vi "Grid_Save_STS_test.vi"(9 "load":u16(ring) items=["numerical_-1V->2V", "numerical_-20mV->20mV", "numerical_-2V->2.2V", "lockin_-20mV->20mV", "lockin_-25mV->25mV", "test", "lockin_highRes_20mV_-20mV", "lockin_slow", "Lock_in_DCA_1.5V->-50mV", "Long_MgPc_lockin_-1->1V", "MgPc_long_lockin", "lockin_slow_-1_2", "MgPc_long_lockin2", "Quick_Lockin"], 10 "stop":bool, 11 "Load":bool) -> (3 "STSTypes []":string[](array[string]))   [LabVIEW 2014]
uses:
  <userlib>/Nanonis Prog Interface V5/Nanonis Prog Interface.lvlib
panel:
  out "loaded":i32
  out "data":T1(array[cluster])
  in  "Save parameters":bool
  in  "Save As":string
  in  "STSparameters":T2 {"End value (V)" min=-10 max=10 format="%#_6p"; "Start value (V)" min=-10 max=10 format="%#_6p"; "End of Sweep"."Z control time (s)" min=0 max=10 step=0.0001 format="%.3p"; "End of Sweep"."End settling time (s)" step=0.0001 format="%.3p"; "Sweep Timing"."Integration time (s)" min=0 max=20 step=0.0001 format="%.3p"; "Sweep Timing"."Settling time (s)" step=0.0001 format="%.3p"; "Sweep Timing"."Max. slew rate (V/s)" format="%.3p"; "Initialization"."Initial settling time (s)" step=0.0001 format="%.3p"; "Initialization"."Z offset (m)" format="%.3p"; "Initialization"."Z averaging time (s)" min=0 max=10 step=0.0001 format="%.3p"; "Amplitude (mod. signal unit)" format="%#_6p"}
  # "make sure\nLockin is activated\nin Advanced Settings"
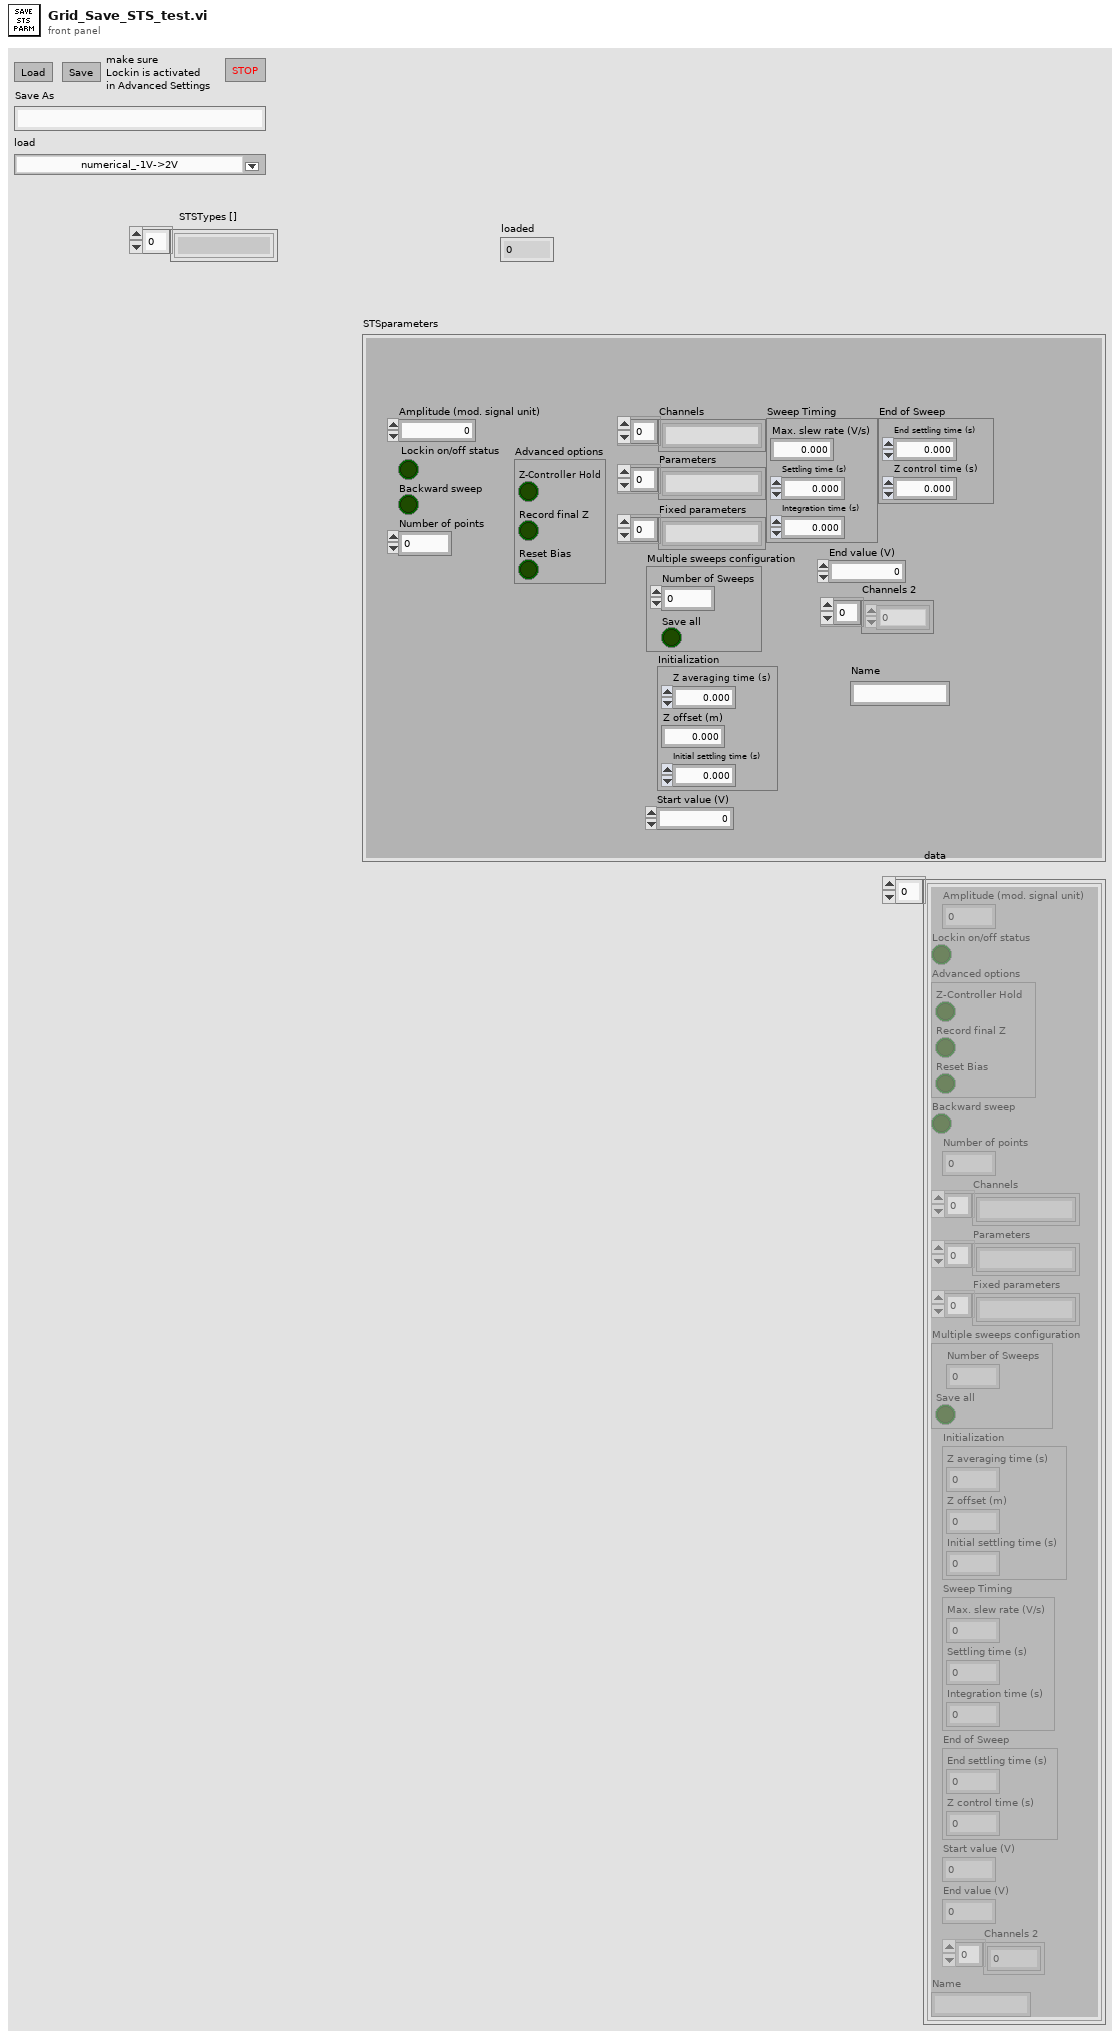
[diagram p1: front panel]
types:
  T1 = cluster{"Amplitude (mod. signal unit)":sgl, "Lockin on/off status":bool, "Advanced options":cluster{"Z-Controller Hold":bool, "Record final Z":bool, "Reset Bias":bool}, "Backward sweep":bool, "Number of points":i32, "Channels":string[], "Parameters":string[], "Fixed parameters":string[], "Multiple sweeps configuration":cluster{"Number of Sweeps":i32, "Save all":bool}, "Initialization":cluster{"Z averaging time (s)":sgl, "Z offset (m)":sgl, "Initial settling time (s)":sgl}, "Sweep Timing":cluster{"Max. slew rate (V/s)":sgl, "Settling time (s)":sgl, "Integration time (s)":sgl}, "End of Sweep":cluster{"End settling time (s)":sgl, "Z control time (s)":sgl}, "Start value (V)":sgl, "End value (V)":sgl, "Channels 2":i32[], "Name":string}[]
  T2 = cluster{"Amplitude (mod. signal unit)":sgl, "Lockin on/off status":bool, "Advanced options":cluster{"Z-Controller Hold":bool, "Record final Z":bool, "Reset Bias":bool}, "Backward sweep":bool, "Number of points":i32, "Channels":string[], "Parameters":string[], "Fixed parameters":string[], "Multiple sweeps configuration":cluster{"Number of Sweeps":i32, "Save all":bool}, "Initialization":cluster{"Z averaging time (s)":sgl, "Z offset (m)":sgl, "Initial settling time (s)":sgl}, "Sweep Timing":cluster{"Max. slew rate (V/s)":sgl, "Settling time (s)":sgl, "Integration time (s)":sgl}, "End of Sweep":cluster{"End settling time (s)":sgl, "Z control time (s)":sgl}, "Start value (V)":sgl, "End value (V)":sgl, "Channels 2":i32[], "Name":string}
  T3 = cluster{"Save all":enum16{"no change", "on", "off"}, "Number of Sweeps (0=no change)":i32}
  T4 = cluster{"Z-Controller Hold":bool, "Record final Z":bool, "Reset Bias":bool}
  T5 = cluster{"Z averaging time (s)":sgl, "Z offset (m)":sgl, "Initial settling time (s)":sgl}
  T6 = cluster{"Max. slew rate (V/s)":sgl, "Settling time (s)":sgl, "Integration time (s)":sgl}
  T7 = cluster{"End settling time (s)":sgl, "Z control time (s)":sgl}
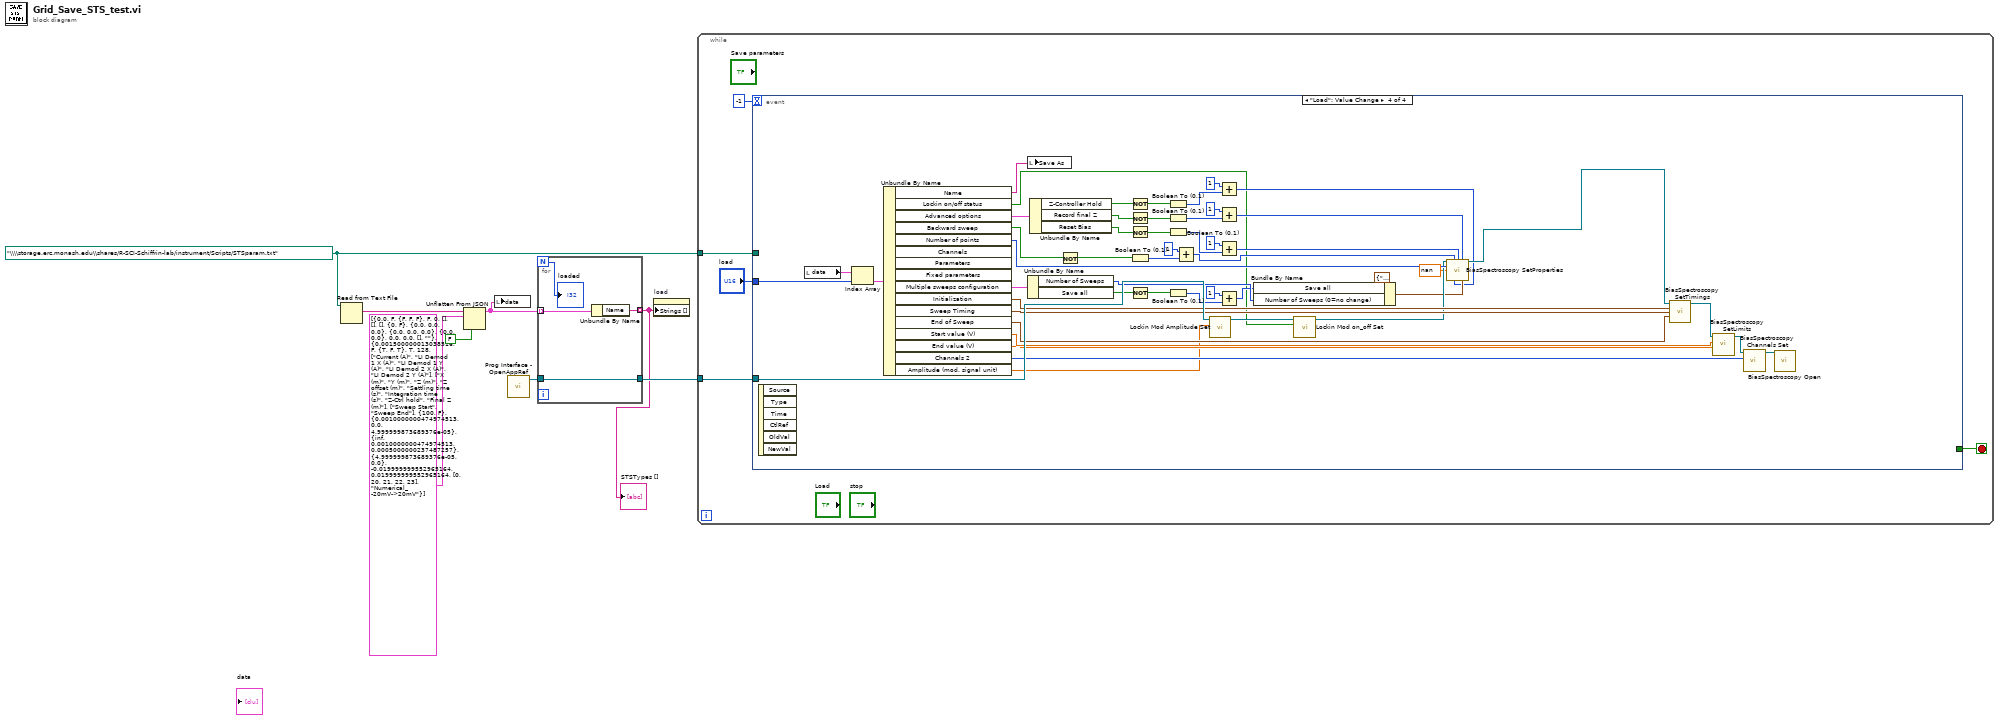
[diagram p0: block diagram]
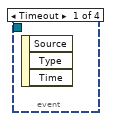
[diagram p2: hidden frame]
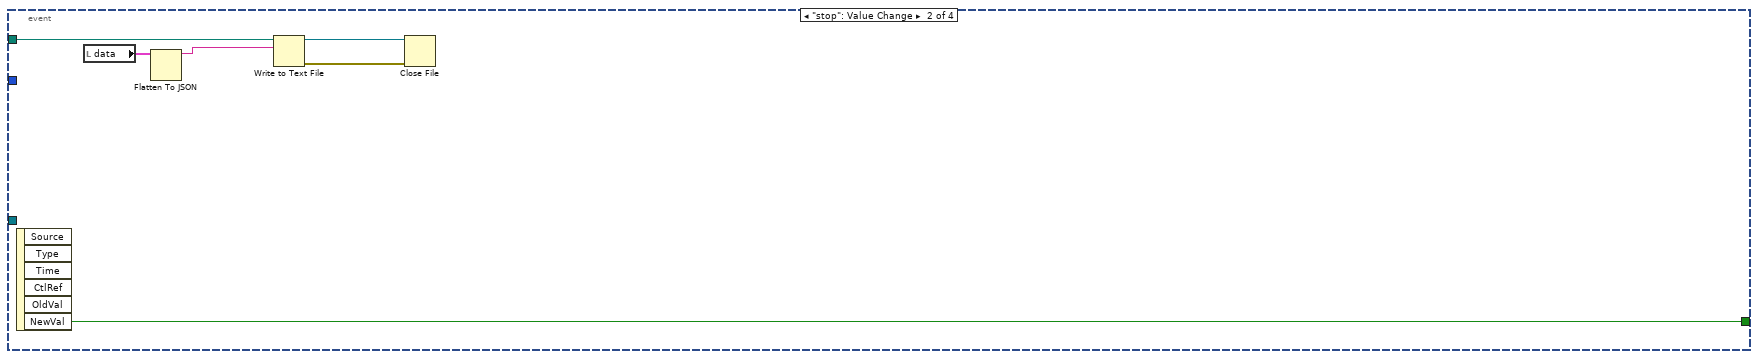
[diagram p3: hidden frame]
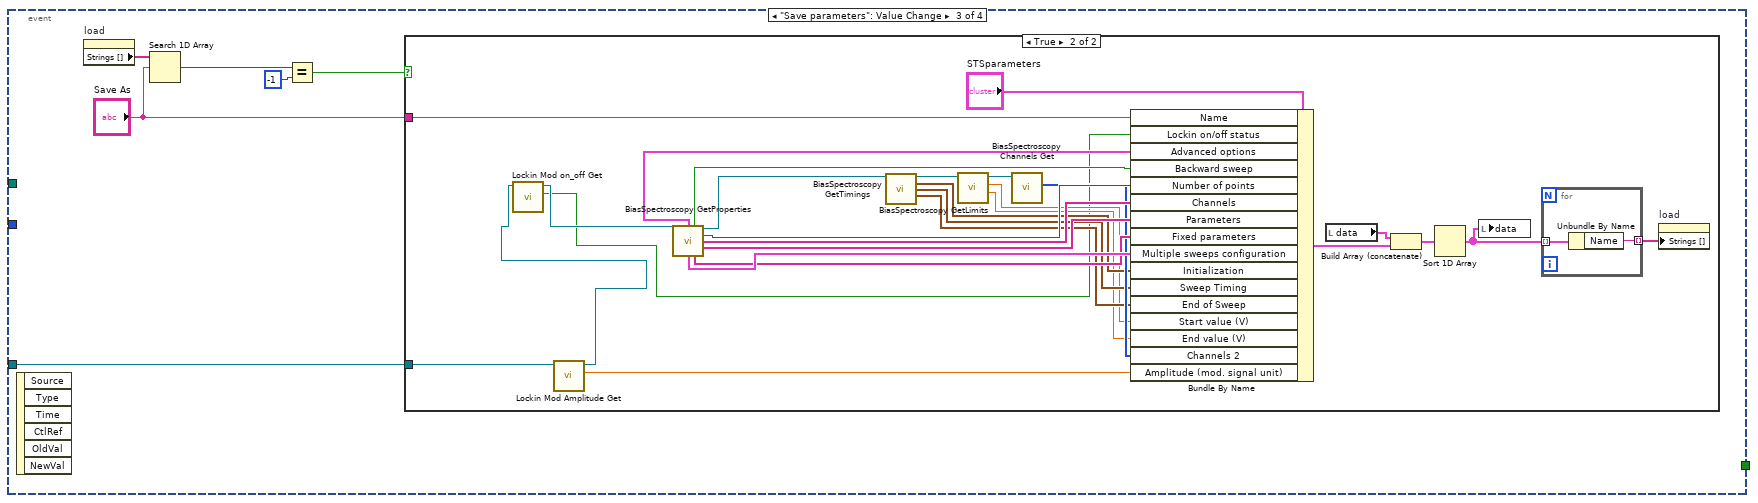
[diagram p4: hidden frame]
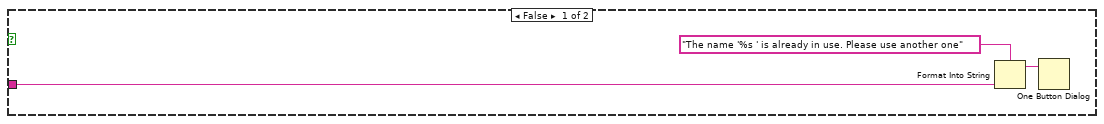
[diagram p5: hidden frame]
diagram:
  w8 = path "\\\\storage.erc.monash.edu\\shares/R-SCI-Schiffrin-lab/instrument/Scripts/STSparam.txt" ("file (use dialog)")
  n1 = Read from Text File(file (use dialog)=w8) -> (text=w7:string)  [unwired: 3 in, 3 out]
  n2 = Unflatten From JSON(JSON string=w7, type and defaults=T1 [{"Amplitude (mod. signal unit)"=0.0, "Lockin on/off status"=FALSE, "Advanced options"={"Z-Controller Hold"=FALSE, "Record final Z"=FALSE, "Reset Bias"=FALSE}, "Backward sweep"=FALSE, "Number of points"=0, "Channels"=[], "Parameters"=[], "Fixed parameters"=[], "Multiple sweeps configuration"={"Number of Sweeps"=0, "Save all"=FALSE}, "Initialization"={"Z averaging time (s)"=0.0, "Z offset (m)"=0.0, "Initial settling time (s)"=0.0}, "Sweep Timing"={"Max. slew rate (V/s)"=0.0, "Settling time (s)"=0.0, "Integration time (s)"=0.0}, "End of Sweep"={"End settling time (s)"=0.0, "Z control time (s)"=0.0}, "Start value (V)"=0.0, "End value (V)"=0.0, "Channels 2"=[], "Name"=""}, {"Amplitude (mod. signal unit)"=0.0015, "Lockin on/off status"=FALSE, "Advanced options"={"Z-Controller Hold"=TRUE, "Record final Z"=FALSE, "Reset Bias"=TRUE}, "Backward sweep"=TRUE, "Number of points"=128, "Channels"=["Current (A)", "LI Demod 1 X (A)", "LI Demod 1 Y (A)", "LI Demod 2 X (A)", "LI Demod 2 Y (A)"], "Parameters"=["X (m)", "Y (m)", "Z (m)", "Z offset (m)", "Settling time (s)", "Integration time (s)", "Z-Ctrl hold", "Final Z (m)"], "Fixed parameters"=["Sweep Start", "Sweep End"], "Multiple sweeps configuration"={"Number of Sweeps"=100, "Save all"=FALSE}, "Initialization"={"Z averaging time (s)"=0.001, "Z offset (m)"=0.0, "Initial settling time (s)"=5e-05}, "Sweep Timing"={"Max. slew rate (V/s)"=inf, "Settling time (s)"=0.001, "Integration time (s)"=0.0005}, "End of Sweep"={"End settling time (s)"=5e-05, "Z control time (s)"=0.0}, "Start value (V)"=-0.02, "End value (V)"=0.02, "Channels 2"=[0, 20, 21, 22, 23], "Name"="Numerical_-20mV->20mV"}] ("data"), default null elements? (F)=FALSE) -> (value=w2:T1)  [unwired: 4 in, 1 out]
  n3 = local write "data"(w2) -> ()
  n4 = call <userlib>:"Prog Interface - OpenAppRef.vi"() -> ("Application reference"=w6:refnum<vi>)  [unwired: 6 in, 1 out]
  n5 = for {
    N -> [w9]
    tunnel: w2 -> [w12] mode=indexing
    tunnel: [w11] -> w1 mode=indexing
    tunnel: w6 -> [w10]
    tunnel: [w10] -> w5
    n6 = Unbundle By Name(w12) -> ("Name"=w11:string)
    "loaded" <- w9
  }
  "STSTypes []" <- w1
  n7 = property on="load" class="Ring (strict)"("Strings []"=w1) -> ()  [unwired: 2 in, 2 out]
  n8 = while {
    tunnel: w5 -> [w17]
    tunnel: w8 -> [w14]
    stop <- w15 stop-if-true
    n9 = event shown="[3] \"Load\": Value Change" {
      selector: _ -> [_ _ _ _]
      dyn-events: _ -> [_ _ _ _]
      timeout: -1 -> [_ _ _ _]
      tunnel: w17 -> [_ _ w29 w111]
      tunnel: "load" -> [_ _ _ w75]
      tunnel: [_ w23 _ _] -> w15
      tunnel: w14 -> [_ w19 _ _]
      event Timeout {
        n10 = event-data() -> ()  [unwired: 1 in, 3 out]
      }
      event "stop": Value Change {
        n11 = event-data() -> ("NewVal"=w23:bool)  [unwired: 1 in, 5 out]
        n12 = local read "data"() -> (w18:T1)
        n13 = Flatten To JSON(anything=w18) -> (JSON string=w22:string)  [unwired: 2 in, 1 out]
        n14 = Write to Text File(file (use dialog)=w19, text=w22) -> (refnum out=w20:refnum<file>, error out=w21:errorcluster)  [unwired: 2 in, 1 out]
        n15 = Close File(refnum=w20, error in=w21) -> ()  [unwired: 2 out]
      }
      event "Save parameters": Value Change {
        n16 = event-data() -> ()  [unwired: 1 in, 6 out]
        n17 = property on="load" class="Ring (strict)"() -> ("Strings []"=w28:string[])  [unwired: 2 in, 2 out]
        n18 = Search 1D Array(1D array=w28, element="Save As") -> (index of element=w26:i32)  [unwired: 1 in]
        n19 = Equal?(x=w26, y=-1) -> (x = y?=w24:bool)
        n20 = case shown="True" w24 {
          tunnel: w29 -> [_ w44]
          tunnel: "Save As" -> [w32 w37]
          frame False {
            n21 = Format Into String(format string="The name '%s ' is already in use. Please use another one", w32) -> (resulting string=w30:string)  [unwired: 2 in, 1 out]
            n22 = One Button Dialog(message=w30) -> ()  [unwired: 1 in, 1 out]
          }
          frame True {
            n23 = call <userlib>:"Lockin Mod Amplitude Get.vi"("Application ref in"=w44) -> ("Amplitude (mod. signal unit)"=w41:sgl, "Application ref out"=w35:refnum<vi>)  [unwired: 8 in, 1 out]
            n24 = call <userlib>:"Lockin Mod on_off Get.vi"("Application ref in"=w35) -> ("Lockin on/off status"=w33:bool, "Application ref out"=w34:refnum<vi>)  [unwired: 8 in, 1 out]
            n25 = call <userlib>:"BiasSpectroscopy GetProperties.vi"("Application ref in"=w34) -> ("Advanced options"=w36:T4, "Backward sweep"=w52:bool, "Application ref out"=w51:refnum<vi>, "Number of points"=w58:i32, "Channels"=w57:string[], "Parameters"=w56:string[], "Multiple sweeps configuration"=w55:cluster{"Number of Sweeps":i32, "Save all":bool}, "Fixed parameters"=w54:string[])  [unwired: 6 in, 1 out]
            n26 = call <userlib>:"BiasSpectroscopy GetTimings.vi"("Application ref in"=w51) -> ("Application ref out"=w59:refnum<vi>, "Initialization"=w50:T5, "Sweep Timing"=w48:T6, "End of Sweep"=w49:T7)  [unwired: 10 in, 1 out]
            n27 = call <userlib>:"BiasSpectroscopy GetLimits.vi"("Application ref in"=w59) -> ("End value (V)"=w46:sgl, "Start value (V)"=w47:sgl, "Application ref out"=w60:refnum<vi>)  [unwired: 5 in, 1 out]
            n28 = call <userlib>:"BiasSpectroscopy Channels Get.vi"("Application ref in"=w60) -> ("Channels"=w53:i32[])  [unwired: 8 in, 2 out]
            n29 = Bundle By Name(cluster="STSparameters", "Name"=w37, "Lockin on/off status"=w33, "Advanced options"=w36, "Backward sweep"=w52, "Number of points"=w58, "Channels"=w57, "Parameters"=w56, "Fixed parameters"=w54, "Multiple sweeps configuration"=w55, "Initialization"=w50, "Sweep Timing"=w48, "End of Sweep"=w49, "Start value (V)"=w47, "End value (V)"=w46, "Channels 2"=w53, "Amplitude (mod. signal unit)"=w41) -> (w45:T2)
            n30 = local read "data"() -> (w42:T1)
            n31 = Build Array (concatenate)(w42, w45) -> (w40:T1)
            n32 = Sort 1D Array(array=w40) -> (sorted array=w39:T1)
            n33 = local write "data"(w39) -> ()
            n34 = for {
              tunnel: w39 -> [w62] mode=indexing
              tunnel: [w61] -> w38 mode=indexing
              n35 = Unbundle By Name(w62) -> ("Name"=w61:string)
            }
            n36 = property on="load" class="Ring (strict)"("Strings []"=w38) -> ()  [unwired: 2 in, 2 out]
          }
        }
      }
      event "Load": Value Change {
        n37 = event-data() -> ()  [unwired: 1 in, 6 out]
        n38 = local read "data"() -> (w113:T1)
        n39 = Index Array(array=w113, index=w75) -> (element=w112:T2)
        n40 = Unbundle By Name(w112) -> ("Name"=w73:string, "Lockin on/off status"=w63:bool, "Advanced options"=w99:T4, "Backward sweep"=w98:bool, "Number of points"=w101:i32, "Multiple sweeps configuration"=w100:cluster{"Number of Sweeps":i32, "Save all":bool}, "Initialization"=w102:T5, "Sweep Timing"=w103:T6, "End of Sweep"=w104:T7, "Start value (V)"=w106:sgl, "End value (V)"=w105:sgl, "Channels 2"=w107:i32[], "Amplitude (mod. signal unit)"=w74:sgl)  [unwired: 3 out]
        n41 = local write "Save As"(w73) -> ()
        n42 = Unbundle By Name(w100) -> ("Number of Sweeps"=w86:i32, "Save all"=w82:bool)
        n43 = Unbundle By Name(w99) -> ("Z-Controller Hold"=w91:bool, "Record final Z"=w90:bool, "Reset Bias"=w87:bool)
        n44 = Not(x=w98) -> (.not. x?=w78:bool)
        n45 = Not(x=w91) -> (.not. x?=w77:bool)
        n46 = Not(x=w90) -> (.not. x?=w80:bool)
        n47 = Not(x=w87) -> (.not. x?=w79:bool)
        n48 = Boolean To (0,1)(Boolean=w78) -> (0, 1=w97:i16)
        n49 = Not(x=w82) -> (.not. x?=w76:bool)
        n50 = Boolean To (0,1)(Boolean=w77) -> (0, 1=w93:i16)
        n51 = Boolean To (0,1)(Boolean=w80) -> (0, 1=w95:i16)
        n52 = Boolean To (0,1)(Boolean=w79) -> (0, 1=w89:i16)
        n53 = Boolean To (0,1)(Boolean=w76) -> (0, 1=w85:i16)
        n54 = Add(x=i16 1, y=w97) -> (x+y=w72:i16)
        n55 = call <userlib>:"Lockin Mod Amplitude Set.vi"("Amplitude (mod. signal unit)"=w74, "Application ref in"=w111) -> ("Application ref out"=w110:refnum<vi>)  [unwired: 8 in, 1 out]
        n56 = Add(x=i16 1, y=w93) -> (x+y=w64:i16)
        n57 = Add(x=i16 1, y=w95) -> (x+y=w65:i16)
        n58 = Add(x=i16 1, y=w89) -> (x+y=w69:i16)
        n59 = Add(x=i16 1, y=w85) -> (x+y=w83:i16)
        n60 = Bundle By Name(cluster=T3 {"Save all"=enum."no change", "Number of Sweeps (0=no change)"=0} ("Multiple sweeps config"), "Save all"=w83, "Number of Sweeps (0=no change)"=w86) -> (w67:T3)
        n61 = call <userlib>:"Lockin Mod on_off Set.vi"("Lockin ON/OFF"=w63, "Application ref in"=w110) -> ("Application ref out"=w71:refnum<vi>)  [unwired: 8 in, 1 out]
        n62 = call <userlib>:"BiasSpectroscopy SetProperties.vi"("Application ref in"=w71, "Backward sweep (no change)"=w72, "Reset Bias (no change)"=w69, "Record final Z position"=w65, "Number of points (0=no change)"=w101, "Z offset (m) (NaN=no change)"=sgl nan, "Z-Controller hold (no change)"=w64, "Multiple sweeps config"=w67) -> ("Application ref out"=w70:refnum<vi>)  [unwired: 6 in, 1 out]
        n63 = call <userlib>:"BiasSpectroscopy SetTimings.vi"("Application ref in"=w70, "Initialization (NaN)"=w102, "Sweep Timing (NaN)"=w103, "End of Sweep (NaN)"=w104) -> ("Application ref out"=w109:refnum<vi>)  [unwired: 10 in, 1 out]
        n64 = call <userlib>:"BiasSpectroscopy SetLimits.vi"("End value (V)"=w105, "Start value (V)"=w106, "Application ref in"=w109) -> ("Application ref out"=w108:refnum<vi>)  [unwired: 5 in, 1 out]
        n65 = call <userlib>:"BiasSpectroscopy Channels Set.vi"("Channels"=w107, "Application ref in"=w108) -> ("Application ref out"=w81:refnum<vi>)  [unwired: 8 in, 1 out]
        n66 = call <userlib>:"BiasSpectroscopy Open.vi"("Application ref in"=w81) -> ()  [unwired: 13 in, 2 out]
      }
    }
  }
